vi "Prepare remote file URI.vi"(8 "error in (no error)":errorcluster, 10 "Remote path":string, 11 "WebDAV in":refnum<class "WebDAV.lvclass">) -> (0 "error out":errorcluster, 2 "Remote file URI":string, 3 "WebDAV out":refnum<class "WebDAV.lvclass">)   [LabVIEW 2015, in "RT Management.lvlib" / "WebDAV.lvclass"]
doc: "Takes a remote path and returns the full file URI, which contains the required target prefix.\n\nExample: \"home/lvuser/natinst/bin\" -> \"http://VM-9068-01/files/home/lvuser/natinst/bin\""
uses:
  WebDAV.lvclass
  File Transfer Behavior/File Transfer Behavior.lvclass/File Transfer Behavior.ctl
  File Transfer Behavior/Get Address.vi
  File Transfer Behavior/File Transfer Behavior.lvclass
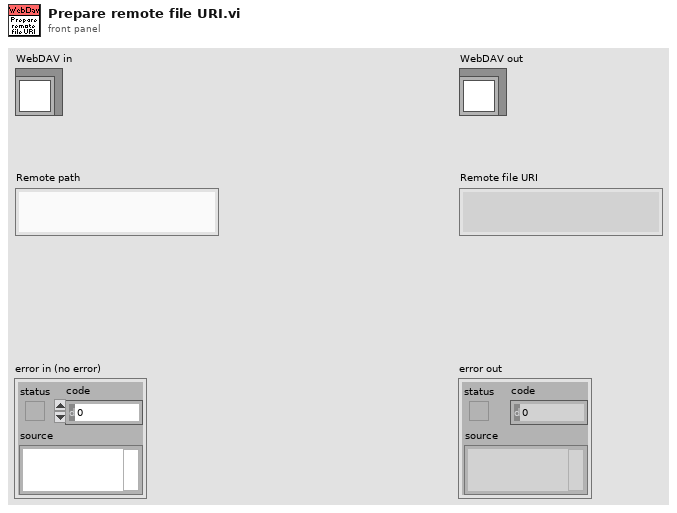
[diagram p1: front panel]
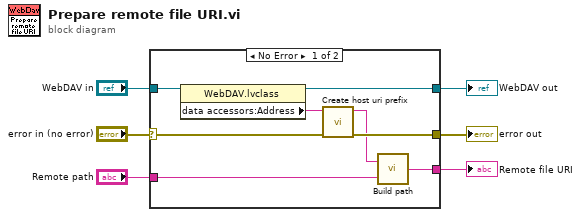
[diagram p0: block diagram]
diagram:
  n1 = case shown="No Error" "error in (no error)" {
    selector: "error in (no error)" -> [w9 w16]
    tunnel: [w11 w16] -> w5
    tunnel: [w10 w15] -> w3
    tunnel: "WebDAV in" -> [w12 w15]
    tunnel: "Remote path" -> [w13 _]
    tunnel: [w14 _] -> w1
    frame No Error {
      n2 = property class="WebDAV.lvclass"(reference=w12) -> (reference out=w10:refnum<class "WebDAV.lvclass">, "data accessors:Address"=w8:string)  [unwired: 1 in, 1 out]
      n3 = call "Create host uri prefix.vi"("error in (no error)"=w9, "address"=w8) -> ("error out"=w11:errorcluster, "host uri prefix"=w7:string)  [unwired: 8 in]
      n4 = call "Build path.vi"("Relative path"=w13, "Base path"=w7) -> ("Resulting path"=w14:string)
    }
    frame Error {
    }
  }
  "error out" <- w5
  "WebDAV out" <- w3
  "Remote file URI" <- w1
